vi "test.vi"() -> ()   [LabVIEW 2021]
uses:
  DoublyNode/DoublyNode.lvclass
  IDoublyNode/IDoublyNode.lvclass
panel:
  out "x = y? 2":bool
  out "x = y?":bool
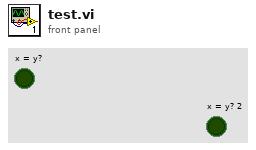
[diagram p1: front panel]
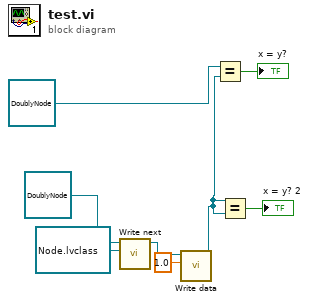
[diagram p0: block diagram]
diagram:
  n1 = call-dynamic "Write next.vi"("next"=refnum<data-value> refnum, "DoublyNode in"=refnum<class "DoublyNode.lvclass"> refnum ("DoublyNode.lvclass")) -> ("DoublyNode out"=w3:refnum<class "DoublyNode.lvclass">)  [unwired: 8 in, 1 out]
  n2 = call-dynamic "Write data.vi"("data"=1.0, "DoublyNode in"=w3) -> ("DoublyNode out"=w2:refnum<class "DoublyNode.lvclass">)  [unwired: 8 in, 1 out]
  n3 = Equal?(x=refnum<class "DoublyNode.lvclass"> refnum ("DoublyNode.lvclass"), y=w2) -> (x = y?=→"x = y?":bool)
  n4 = Equal?(x=w2, y=w2) -> (x = y?=→"x = y? 2":bool)
